vi "test.vi"() -> ()   [LabVIEW 2024, in "Ball-Ball.lvclass"]
doc: "MIT Licence\nCopyright (c) 2024 David Grollier"
uses:
  Ball-Ball.lvclass
  Type Def/Velocity.ctl
  Type Def/Coordinates.ctl
  <vilib>/Utility/miscctls.llb/LVBoundsTypeDef.ctl
  Game Componants/Game Board Component/Movable/Flying Saucer/Flying Saucer.lvclass
  <vilib>/Analysis/7linalg.llb/Subspaces Angle (1D).vi
  Game Componants/Game Board Component/Movable/Movable.lvclass
  Game Componants/Game Board/Game Board.lvclass
  <vilib>/Analysis/NI_AAL_LinAlg.lvlib
panel:
  out "x-y":T1
  out "In Range?":bool
  out "angle":dbl
  out "lower angle":dbl
  out "upper angle":dbl
  out "Velocity player":T1
  out "Velocity target":T1
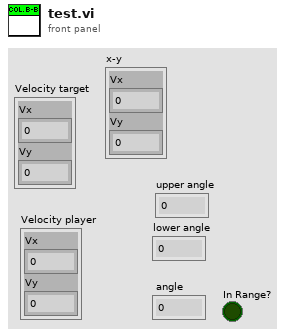
[diagram p1: front panel]
types:
  T1 = typedef "Velocity.ctl" = cluster{"Vx":dbl, "Vy":dbl}
  T2 = typedef "Coordinates.ctl" = cluster{"x":dbl, "y":dbl}
  T3 = typedef "LVBoundsTypeDef.ctl" = cluster{"Width":u32, "Height":u32}
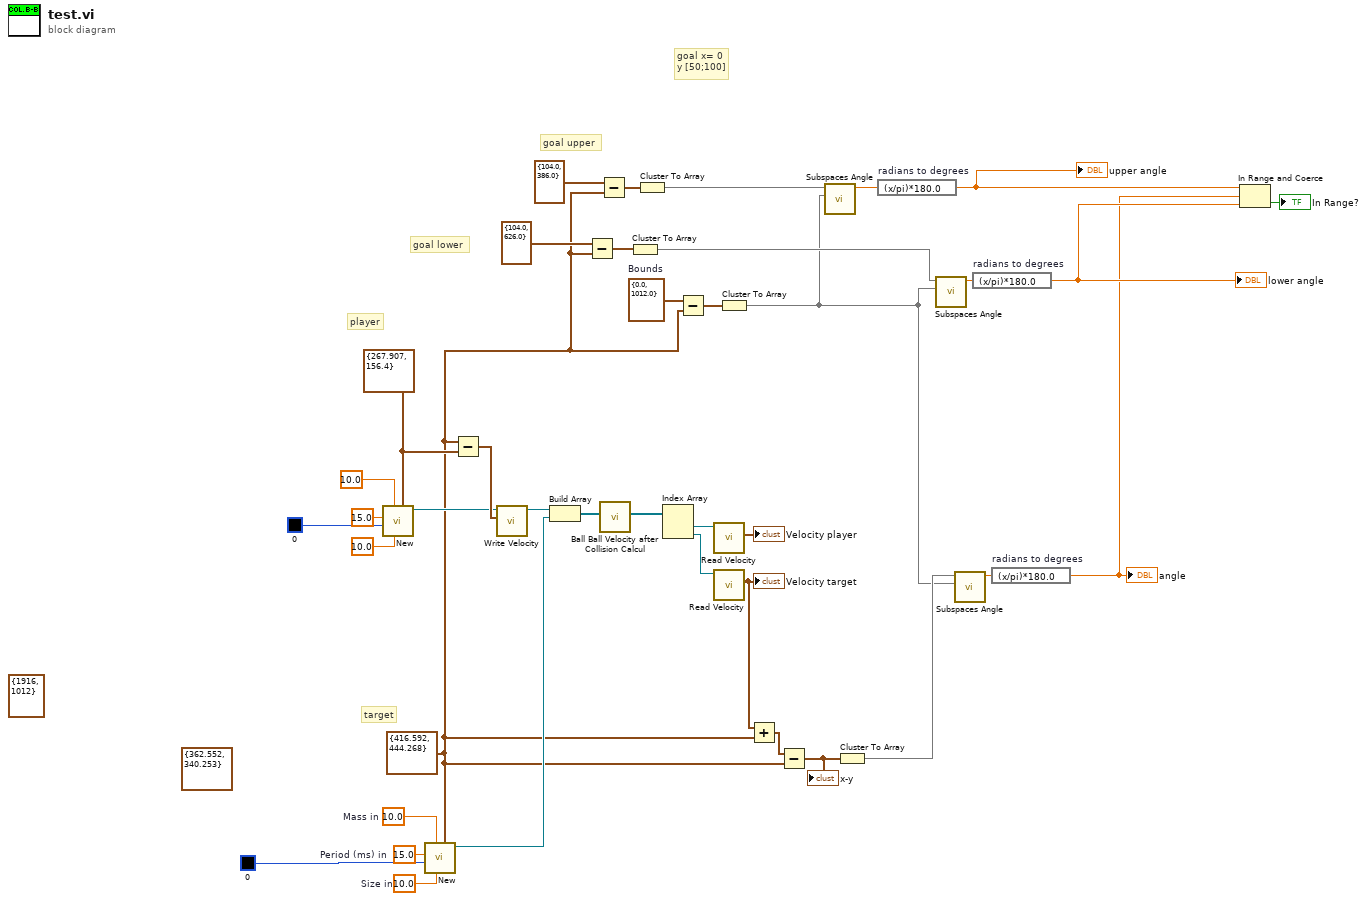
[diagram p0: block diagram]
diagram:
  (unwired) T2 {"x"=362.552, "y"=340.253} ("Coordinates in")
  (unwired) T3 {"Width"=1916, "Height"=1012} ("Bounds in")
  w18 = T2 {"x"=0.0, "y"=1012.0}  # Bounds
  w35 = 10.0  # Size in
  w33 = 15.0  # Period (ms) in
  w32 = 10.0  # Mass in
  w1 = T2 {"x"=416.592, "y"=444.268} ("Coordinates in")
  w17 = T2 {"x"=267.907, "y"=156.4} ("Coordinates in")
  # "goal lower"
  # "goal upper"
  # "goal x= 0\ny [50;100]"
  # "player"
  # "target"
  n1 = call "New.vi"("Coordinates in"=w17, "Size in"=10.0, "Mass in"=10.0, "color in"=u32 0, "Period (ms) in"=15.0) -> ("Flying Saucer out"=w30:refnum<class "Flying Saucer.lvclass">)  [unwired: 6 in]
  n2 = call "New.vi"("Coordinates in"=w1, "Size in"=w35, "Mass in"=w32, "color in"=u32 0, "Period (ms) in"=w33) -> ("Flying Saucer out"=w28:refnum<class "Flying Saucer.lvclass">)  [unwired: 6 in]
  n3 = Subtract(x=w1, y=w17) -> (x-y=w31:T2)
  n4 = call "Write Velocity.vi"("Velocity"=w31, "Movable in"=w30) -> ("Movable out"=w29:refnum<class "Flying Saucer.lvclass">)  [unwired: 9 in]
  n5 = Build Array(w29, w28) -> (w27:refnum<class "Flying Saucer.lvclass">[])
  n6 = Subtract(x=T2 {"x"=104.0, "y"=626.0} ("Coordinates in"), y=w1) -> (x-y=w16:T2)
  n7 = Subtract(x=T2 {"x"=104.0, "y"=386.0} ("Coordinates in"), y=w1) -> (x-y=w15:T2)
  n8 = call "Ball Ball Velocity after Collision Calcul.vi"("Movables in"=w27) -> ("Movables out"=w26:refnum<class "Movable.lvclass">[])  [unwired: 10 in]
  n9 = Cluster To Array(cluster=w16) -> (array=w10:dbl[])
  n10 = Cluster To Array(cluster=w15) -> (array=w12:dbl[])
  n11 = Index Array(array=w26) -> (element #1=w24:refnum<class "Movable.lvclass">, element #2=w25:refnum<class "Movable.lvclass">)  [unwired: 2 in]
  n12 = Subtract(x=w18, y=w1) -> (x-y=w14:T2)
  n13 = call-dynamic "Read Velocity.vi"("Movable in"=w24) -> ("Velocity"=→"Velocity player":T1)  [unwired: 10 in]
  n14 = call-dynamic "Read Velocity.vi"("Movable in"=w25) -> ("Velocity"=w22:T1)  [unwired: 10 in]
  "Velocity target" <- w22
  n15 = Cluster To Array(cluster=w14) -> (array=w4:dbl[])
  n16 = Add(x=w22, y=w1) -> (x+y=w21:T1)
  n17 = Subtract(x=w21, y=w1) -> (x-y=w7:T1)
  "x-y" <- w7
  n18 = call-poly <vilib>:"Subspaces Angle.vi"("B"=w4, "A"=w12) -> ("angle"=w13:dbl)  [unwired: 8 in, 1 out]
  n19 = Cluster To Array(cluster=w7) -> (array=w5:dbl[])
  n20 = expression code="(x/pi)*180.0" "radians to degrees"(w13) -> (w9:dbl)
  "upper angle" <- w9
  n21 = call-poly <vilib>:"Subspaces Angle.vi"("B"=w4, "A"=w10) -> ("angle"=w11:dbl)  [unwired: 8 in, 1 out]
  n22 = call-poly <vilib>:"Subspaces Angle.vi"("B"=w4, "A"=w5) -> ("angle"=w6:dbl)  [unwired: 8 in, 1 out]
  n23 = expression code="(x/pi)*180.0" "radians to degrees"(w11) -> (w8:dbl)
  "lower angle" <- w8
  n24 = expression code="(x/pi)*180.0" "radians to degrees"(w6) -> (w3:dbl)
  "angle" <- w3
  n25 = In Range and Coerce(upper limit=w9, x=w3, lower limit=w8) -> (In Range?=→"In Range?":bool)  [unwired: 1 out]
